vi "Reformat.vi"() -> ()   [LabVIEW 2018]
uses:
  <vilib>/Utility/file.llb/Read Delimited Spreadsheet (DBL).vi
  <vilib>/Utility/file.llb/Write Delimited Spreadsheet (string).vi
  <vilib>/Utility/file.llb/Write Delimited Spreadsheet (DBL).vi
panel:
  out "all rows":dbl[][](array[numeric])
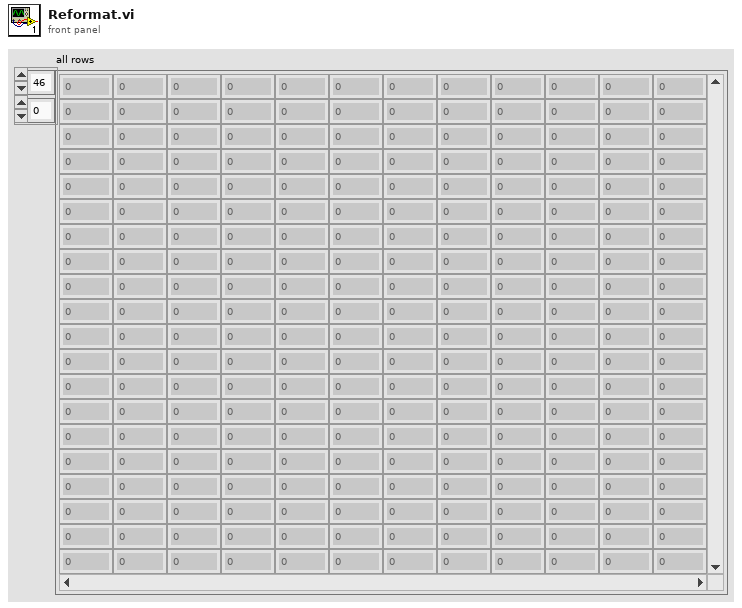
[diagram p1: front panel]
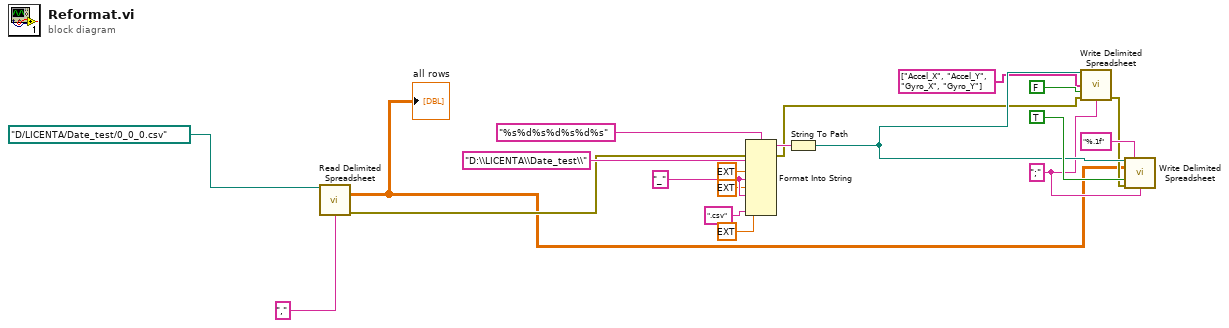
[diagram p0: block diagram]
diagram:
  w10 = "_"
  w15 = ";" ("delimiter (\\t)")
  n1 = call-poly <vilib>:"Read Delimited Spreadsheet.vi"("file path (dialog if empty)"=path "D:/LICENTA/Date_test/0_0_0.csv", "delimiter (\\t)"="," ("delimiter (\\t)")) -> ("all rows"=w1:dbl[][], "error out"=w5:errorcluster)  [unwired: 8 in, 4 out]
  "all rows" <- w1
  n2 = Format Into String(format string="%s%d%s%d%s%d%s", error in=w5, "D:\\LICENTA\\Date_test\\", ext 0.0 ("input 2"), w10, ext 0.0 ("input 4"), w10, ext 0.0 ("input 6"), ".csv" ("input 7")) -> (resulting string=w9:string, error out=w7:errorcluster)  [unwired: 1 in]
  n3 = String To Path(string=w9) -> (path=w16:path)
  n4 = call-poly <vilib>:"Write Delimited Spreadsheet.vi"("file path (dialog if empty)"=w16, "1D data"=string[] ["Accel_X", "Accel_Y", "Gyro_X", "Gyro_Y"] ("Array"), "append to file? (new file:F)"=FALSE, "error in (no error)"=w7, "delimiter (\\t)"=w15) -> ("error out"=w6:errorcluster)  [unwired: 9 in, 1 out]
  n5 = call-poly <vilib>:"Write Delimited Spreadsheet.vi"("file path (dialog if empty)"=w16, "format (%.3f)"="%.1f", "2D data"=w1, "append to file? (new file:F)"=TRUE, "error in (no error)"=w6, "delimiter (\\t)"=w15) -> ()  [unwired: 8 in, 2 out]
